vi "Read Cooler Status.vi"(8 "error in (no error)":errorcluster, 11 "Cooler in":refnum<class "Simulated_Cooler.lvclass">) -> (0 "error out":errorcluster, 1 "temp status":string, 2 "Current temp":i16, 3 "Cooler out":refnum<class "Simulated_Cooler.lvclass">)   [LabVIEW 2018, in "Simulated_Cooler.lvclass"]
uses:
  Simulated_Cooler.lvclass
  Simulated_Cooler.lvclass/Simulated_Cooler.ctl
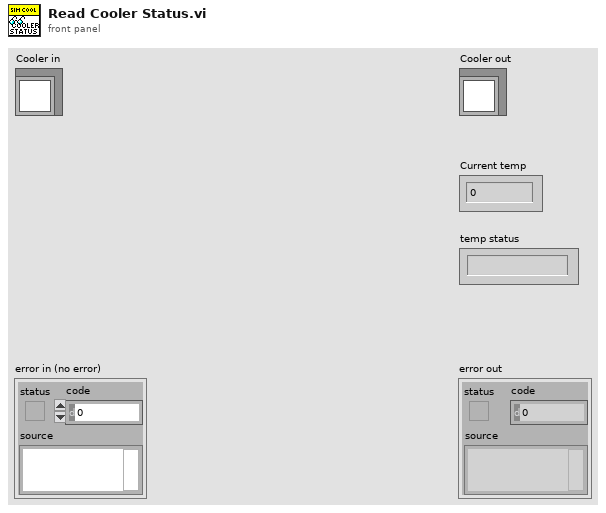
[diagram p1: front panel]
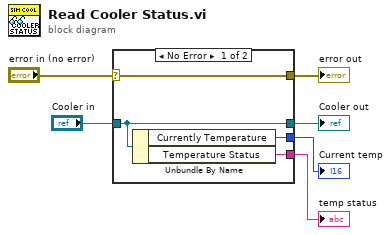
[diagram p0: block diagram]
diagram:
  n1 = case shown="No Error" "error in (no error)" {
    selector: "error in (no error)" -> [w10 w12]
    tunnel: [w10 w12] -> w5
    tunnel: [w9 w11] -> w3
    tunnel: "Cooler in" -> [w9 w11]
    tunnel: [w8 _] -> w2
    tunnel: [w7 _] -> w1
    frame No Error {
      n2 = Unbundle By Name(w9) -> ("Currently Temperature"=w8:i16, "Temperature Status"=w7:string)
    }
    frame Error {
    }
  }
  "error out" <- w5
  "Cooler out" <- w3
  "temp status" <- w1
  "Current temp" <- w2
